vi "getKeyOrIndex2.vi"(8 "error in (no error)":errorcluster, 9 "before match":string, 10 "previous level cluster":variant, 11 "input string":string) -> (0 "error out":errorcluster, 3 "index out":i32)   [LabVIEW 2015]
uses:
  <vilib>/regexp/Match Regular Expression.xnode
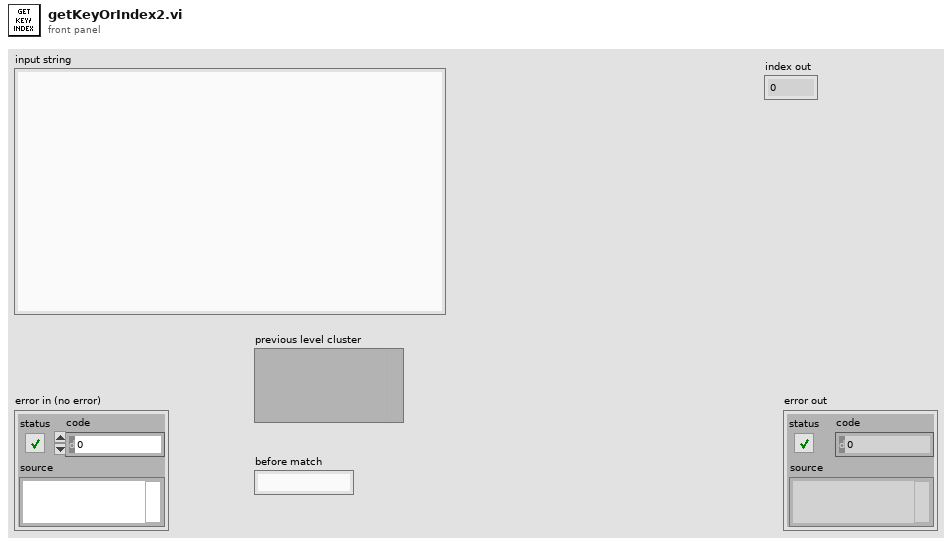
[diagram p1: front panel]
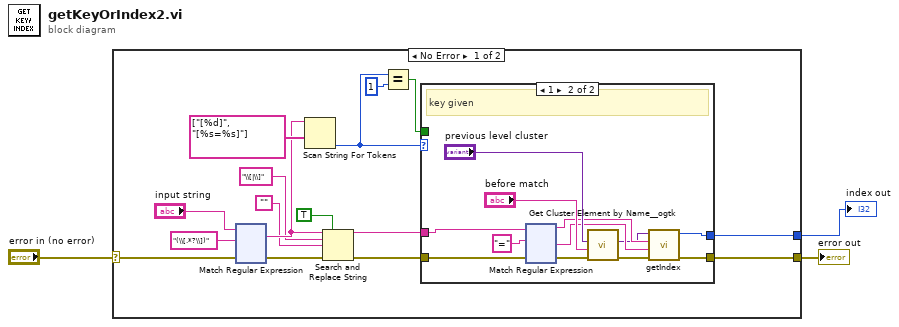
[diagram p0: block diagram]
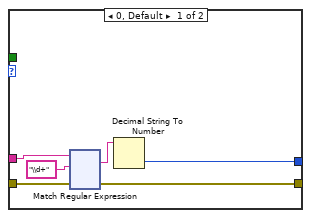
[diagram p2: hidden frame]
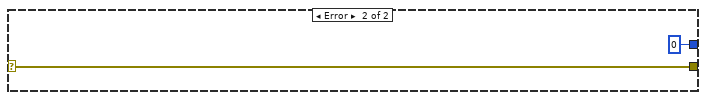
[diagram p3: hidden frame]
diagram:
  n1 = case shown="No Error" "error in (no error)" {
    selector: "error in (no error)" -> [w7 w381]
    tunnel: [w5 w381] -> w2
    tunnel: [w4 0 ("indexOut")] -> w1
    frame No Error {
      n2 = xnode "Match Regular Expression"("input string"="input string", "regular expression"="(\\[.*?\\])", "error in"=w7) -> ("whole match"=w16:string, "error out"=w8:errorcluster)  [unwired: 3 in, 3 out]
      n3 = Scan String For Tokens(7:string[] ["[%d]", "[%s=%s]"] ("operators (none)"), 9:w16) -> (0:w11:i32)  [unwired: 4 in, 3 out]
      n4 = Search and Replace String(replace all?=TRUE ("replace all? (F)"), input string=w16, search string="\\[|\\]", replace string="", error in=w8) -> (result string=w13:string, error out=w9:errorcluster)  [unwired: 3 in, 2 out]
      n5 = Equal?(x=w11, y=1) -> (x = y?=w6:bool)
      n6 = case shown="1" w11 {
        tunnel: w13 -> [w25 w151]
        tunnel: w9 -> [w22 w149]
        tunnel: w6 -> [_ _]
        tunnel: [w21 w143] -> w4
        tunnel: [w20 w140] -> w5
        frame 0, Default {
          n7 = xnode "Match Regular Expression"("input string"=w25, "regular expression"="\\d+", "error in"=w22) -> ("whole match"=w23:string, "error out"=w20:errorcluster)  [unwired: 3 in, 3 out]
          n8 = Decimal String To Number(string=w23) -> (number=w21:i32)  [unwired: 2 in, 1 out]
        }
        frame 1 {
          # "key given"
          n9 = xnode "Match Regular Expression"("input string"=w151, "regular expression"="=", "error in"=w149) -> ("before match"=w146:string, "after match"=w145:string, "error out"=w142:errorcluster)  [unwired: 3 in, 2 out]
          n10 = call <userlib>:"Get Cluster Element by Name__ogtk.vi"("error in (no error)"=w142, "Element Name"="before match", "Cluster"="previous level cluster") -> ("error out"=w141:errorcluster, "VElement"=w144:variant)  [unwired: 6 in, 1 out]
          n11 = call "getIndex.vi"("error in (no error)"=w141, "value"=w145, "key"=w146, "VElement"=w144) -> ("error out"=w140:errorcluster, "indexOut"=w143:i32)  [unwired: 6 in]
        }
      }
    }
    frame Error {
    }
  }
  "error out" <- w2
  "index out" <- w1
